vi "数据查询_数据查询.vi"() -> ()   [LabVIEW 2016]
uses:
  <vilib>/Utility/miscctls.llb/LVPointTypeDef.ctl
  <vilib>/addons/database/_DB Variant To Data/Database Variant To Data.xnode
panel:
  out "确定查询":bool
  out "显示项":string[](array[string])
  out "condition":string
  out "Line Chart":T1(xcontrol)
  in  "数据列表选择框":string(xcontrol)
  out "选中数据表":string
  in  "条件筛选":bool
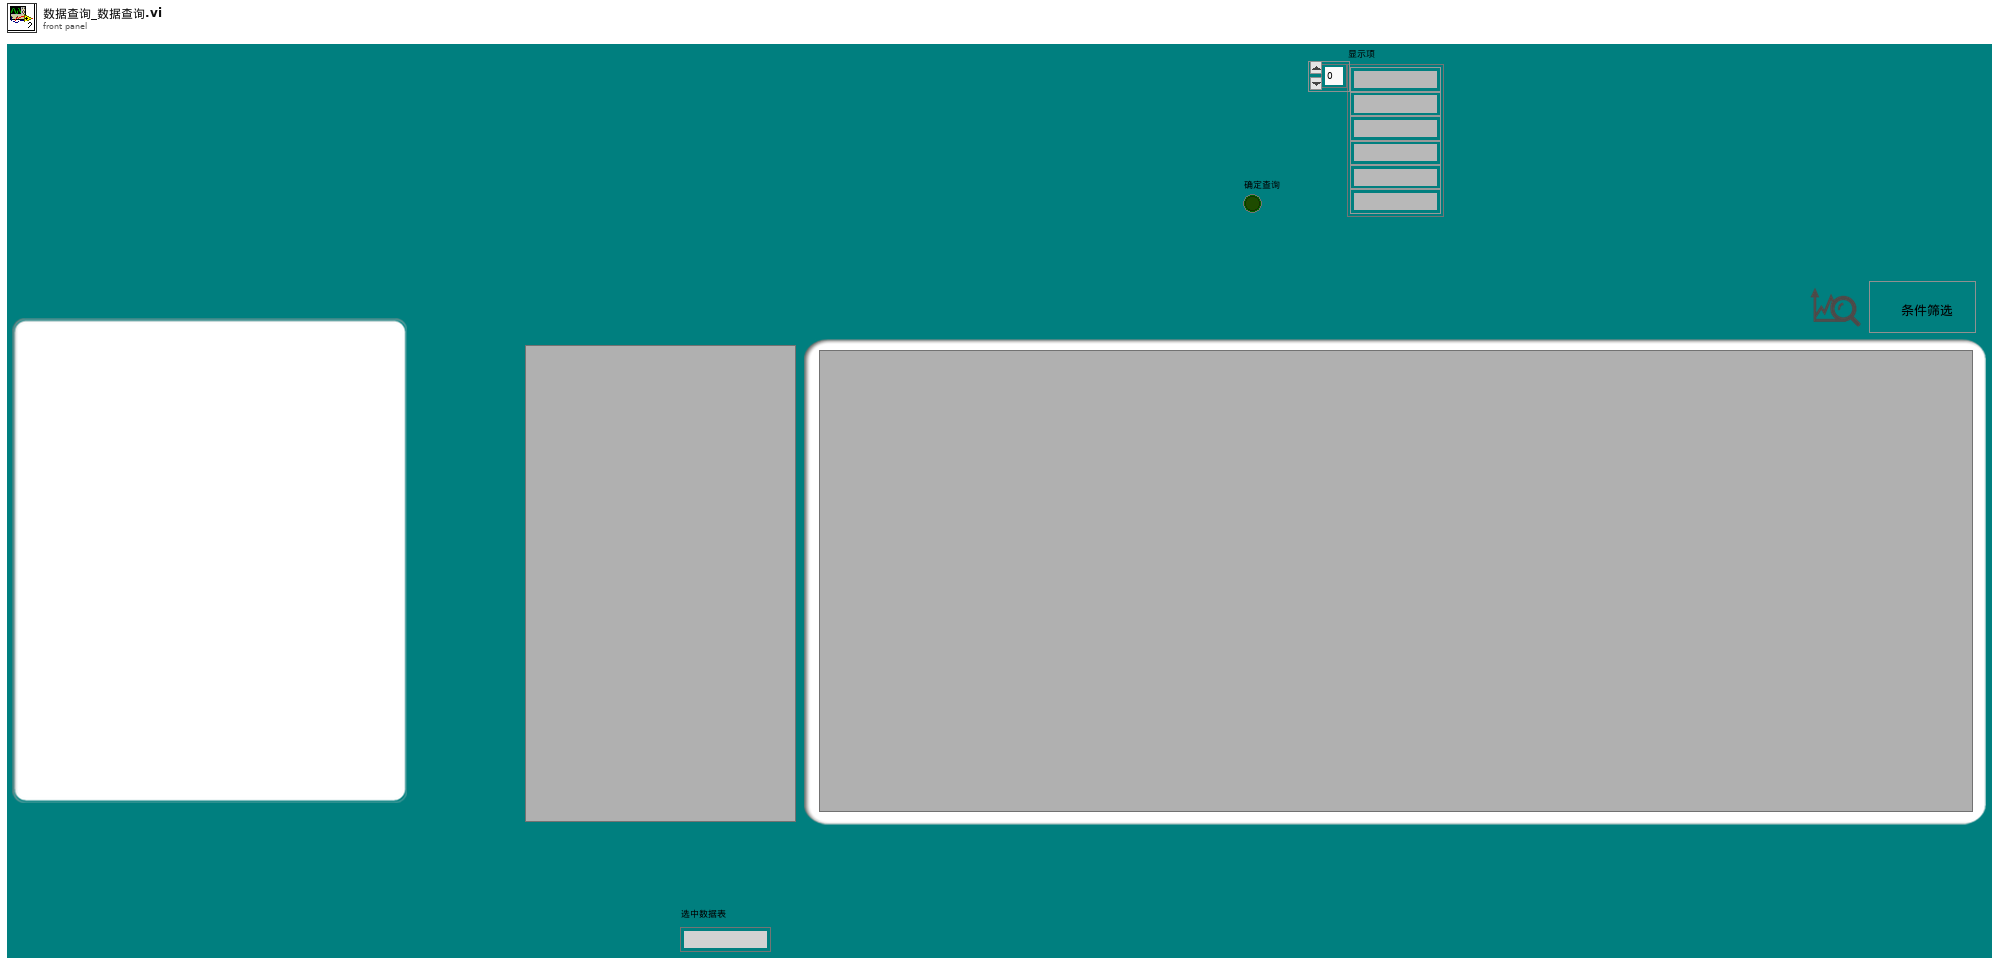
[diagram p1: front panel]
types:
  T1 = cluster{"X-Axis":string[], "Plots":cluster{"Data":dbl[], "Label":string, "Y-Axis":enum16{"Y-Axis 1", "Y-Axis 2", "Y-Axis 3", "Y-Axis 4", "Y-Axis 5", "Y-Axis 6", "Y-Axis 7", "Y-Axis 8", "Y-Axis 9", "Y-Axis 10"}, "Color":u32}[], "Plot Title":string}
  T2 = typedef "LVPointTypeDef.ctl" = cluster{"Horizontal":i16, "Vertical":i16}
  T3 = cluster{"Data":dbl[], "Label":string, "Y-Axis":enum16{"Y-Axis 1", "Y-Axis 2", "Y-Axis 3", "Y-Axis 4", "Y-Axis 5", "Y-Axis 6", "Y-Axis 7", "Y-Axis 8", "Y-Axis 9", "Y-Axis 10"}, "color":u32}
  T4 = cluster{"Data":dbl[], "Label":string, "Y-Axis":enum16{"Y-Axis 1", "Y-Axis 2", "Y-Axis 3", "Y-Axis 4", "Y-Axis 5", "Y-Axis 6", "Y-Axis 7", "Y-Axis 8", "Y-Axis 9", "Y-Axis 10"}, "Color":u32}
  T5 = cluster{"Data":dbl[], "Label":string, "Y-Axis":enum16{"Y-Axis 1", "Y-Axis 2", "Y-Axis 3", "Y-Axis 4", "Y-Axis 5", "Y-Axis 6", "Y-Axis 7", "Y-Axis 8", "Y-Axis 9", "Y-Axis 10"}, "color":u32}[]
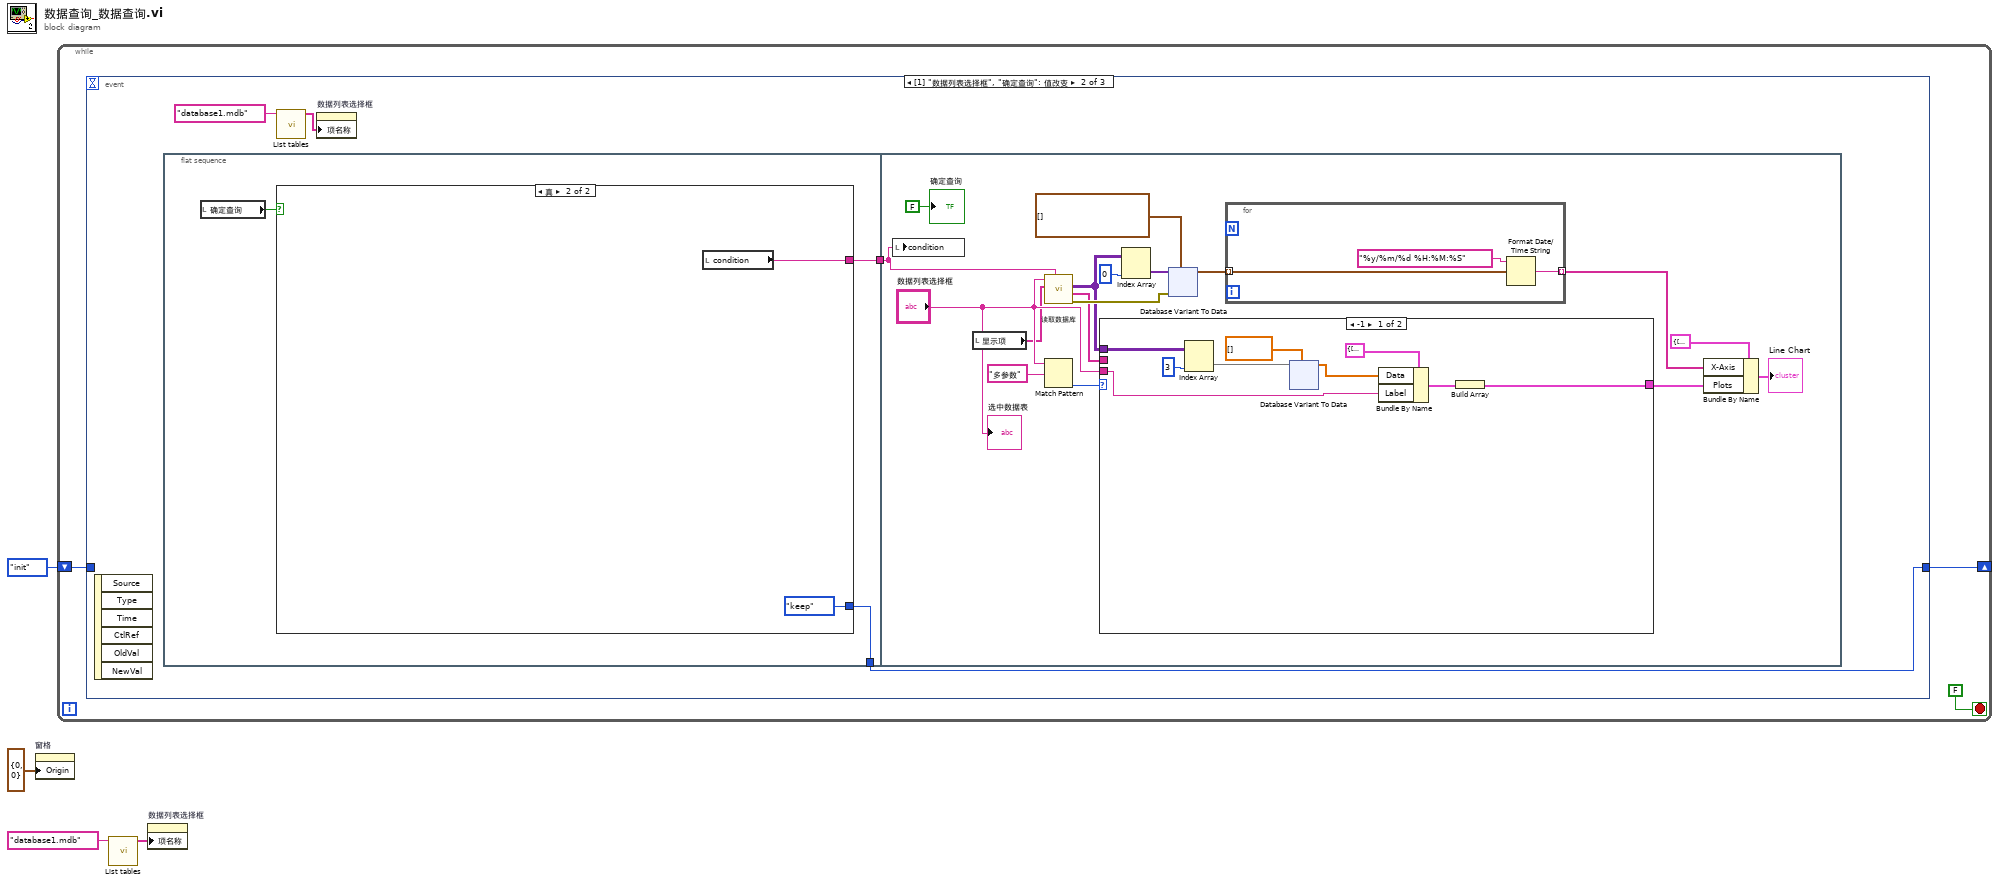
[diagram p0: block diagram]
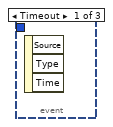
[diagram p2: hidden frame]
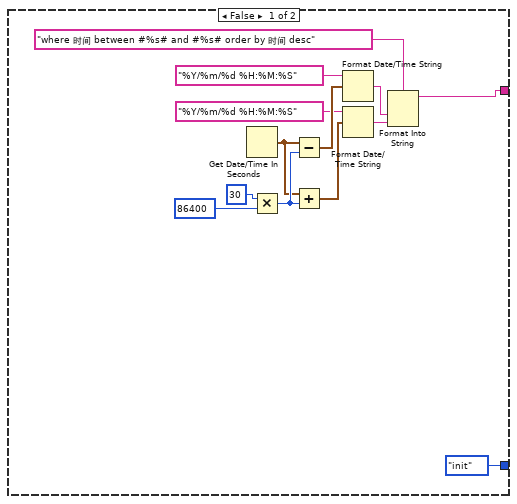
[diagram p3: hidden frame]
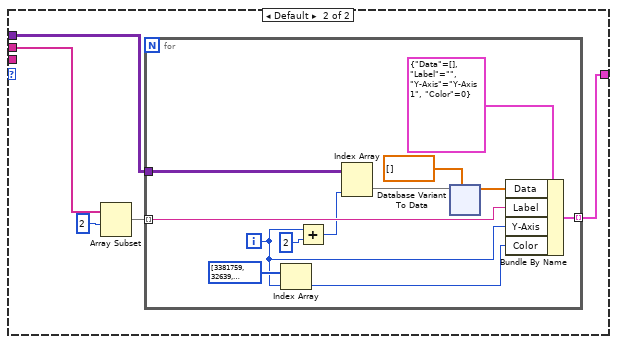
[diagram p4: hidden frame]
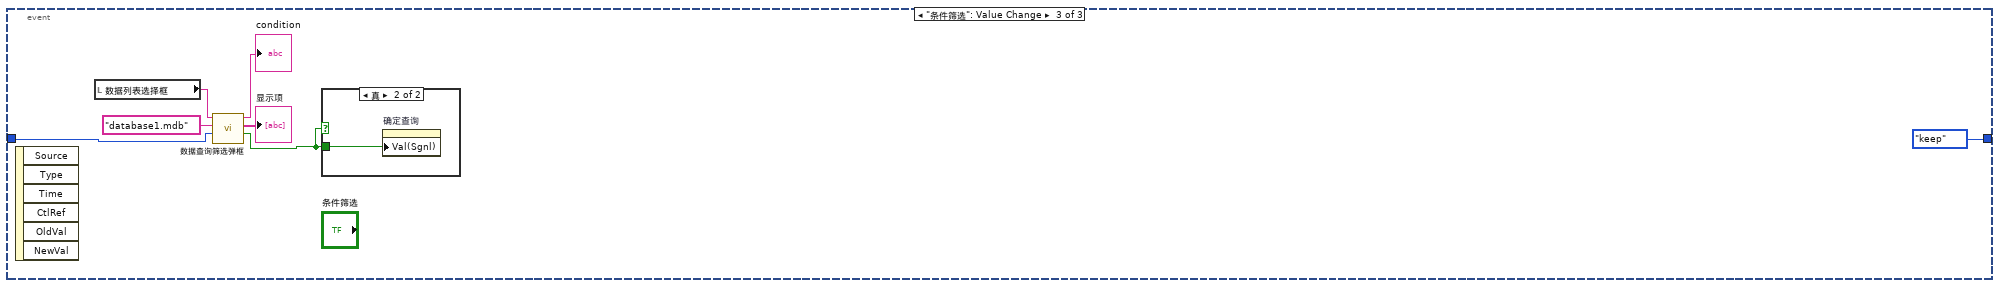
[diagram p5: hidden frame]
diagram:
  n1 = property on="窗格" class="Pane"("Origin"=T2 {"Horizontal"=0, "Vertical"=0} ("原点")) -> ()  [unwired: 2 in, 2 out]
  n2 = while {
    shift-right: [w5] -> _
    shift-left: enum16{"init", "keep"}."init" ("是否初始化") -> [w6]
    stop <- FALSE stop-if-true
    n3 = event shown="[1] \"数据列表选择框\", \"确定查询\": 值改变" {
      selector: _ -> [_ _ _]
      dyn-events: _ -> [_ _ _]
      timeout: _ -> [_ _ _]
      tunnel: w6 -> [_ _ w206]
      tunnel: [_ w8 enum16{"init", "keep"}."keep" ("是否初始化")] -> w5
      event Timeout {
        n4 = event-data() -> ()  [unwired: 1 in, 3 out]
      }
      event "数据列表选择框", "确定查询": Value Change {
        n5 = event-data() -> ()  [unwired: 1 in, 6 out]
        n6 = flat-sequence {
          tunnel: [w13] -> w9
          tunnel: [w12] -> w8
          tunnel: w9 -> [w30]
          frame #0 {
            n7 = local read "确定查询"() -> (w14:bool)
            n8 = case shown="真" w14 {
              tunnel: [w16 w28] -> w13
              tunnel: [enum16{"init", "keep"}."init" ("是否初始化") enum16{"init", "keep"}."keep" ("是否初始化")] -> w12
              frame False {
                n9 = Get Date/Time In Seconds() -> (seconds since 1Jan1904=w17:timestamp)
                n10 = Multiply(x=30, y=86400) -> (x*y=w18:i32)
                n11 = Subtract(x=w17, y=w18) -> (x-y=w24:timestamp)
                n12 = Add(x=w17, y=w18) -> (x+y=w23:timestamp)
                n13 = Format Date/Time String(time format string (%c)="%Y/%m/%d %H:%M:%S" ("时间格式字符串(%c)"), seconds (now)=w24) -> (date/time string=w26:string)  [unwired: 1 in]
                n14 = Format Date/Time String(time format string (%c)="%Y/%m/%d %H:%M:%S" ("时间格式字符串(%c)"), seconds (now)=w23) -> (date/time string=w27:string)  [unwired: 1 in]
                n15 = Format Into String(format string="where 时间 between #%s# and #%s# order by 时间 desc", w26, w27) -> (resulting string=w16:string)  [unwired: 2 in, 1 out]
              }
              frame True {
                n16 = local read "condition"() -> (w28:string)
              }
            }
          }
          frame #1 {
            n17 = local write "condition"(w30) -> ()
            n18 = local read "显示项"() -> (w32:string[])
            n19 = call "读取数据库.vi"("condition"=w30, "显示项"=w32, "组合框"="数据列表选择框") -> ("error out"=w43:errorcluster, "columns"=w35:string[], "data"=w42:variant[][])  [unwired: 5 in, 1 out]
            n20 = Match Pattern(string="数据列表选择框", regular expression="多参数" ("正则表达式")) -> (offset past match=w36:i32)  [unwired: 1 in, 3 out]
            n21 = case shown="-1" w36 {
              tunnel: w42 -> [w55 w98]
              tunnel: [w49 w94] -> w39
              tunnel: "数据列表选择框" -> [w48 _]
              tunnel: w35 -> [_ w97]
              frame -1 {
                n22 = Index Array(array=w55, index (col)=3 ("禁用的索引 (列)")) -> (element=w53:variant[])  [unwired: 1 in]
                n23 = xnode "Database Variant To Data"("database variant"=w53, "type"=sgl[] []) -> ("data"=w51:sgl[])  [unwired: 1 in, 1 out]
                n24 = Bundle By Name(cluster=T3 {"Data"=[], "Label"="", "Y-Axis"=enum."Y-Axis 1", "color"=3381759} ("Plot"), "Data"=w51, "Label"=w48) -> (w50:T3)
                n25 = Build Array(w50) -> (w49:T5)
              }
              frame Default {
                n26 = Array Subset(array=w97, index=2 ("索引")) -> (w95:string[])  [unwired: 1 in]
                n27 = for {
                  tunnel: w98 -> [w110]
                  tunnel: [w106] -> w94 mode=indexing
                  tunnel: w95 -> [w105] mode=indexing
                  i -> [w99]
                  n28 = Index Array(array=u32[] [3381759, 32639, 16744576, 16776960, 16711680, 16860, 8388863, 8404992, 10654332, 12819898], index=w99) -> (element=w101:u32)
                  n29 = Add(x=w99, y=2) -> (x+y=w103:i32)
                  n30 = Index Array(array=w110, index (col)=w103) -> (element=w109:variant[])  [unwired: 1 in]
                  n31 = xnode "Database Variant To Data"("database variant"=w109, "type"=sgl[] []) -> ("data"=w107:sgl[])  [unwired: 1 in, 1 out]
                  n32 = Bundle By Name(cluster=T4 {"Data"=[], "Label"="", "Y-Axis"=enum."Y-Axis 1", "Color"=0} ("Plot"), "Data"=w107, "Label"=w105, "Y-Axis"=w99, "Color"=w101) -> (w106:T4)
                }
              }
            }
            n33 = Index Array(array=w42, index (col)=0 ("禁用的索引 (列)")) -> (element=w45:variant[])  [unwired: 1 in]
            n34 = xnode "Database Variant To Data"("database variant"=w45, "error in (no error)"=w43, "type"=timestamp[] []) -> ("data"=w41:timestamp[])  [unwired: 1 out]
            n35 = for {
              tunnel: w41 -> [w151] mode=indexing
              tunnel: [w150] -> w40 mode=indexing
              n36 = Format Date/Time String(time format string (%c)="%y/%m/%d %H:%M:%S" ("时间格式字符串(%c)"), seconds (now)=w151) -> (date/time string=w150:string)  [unwired: 1 in]
            }
            n37 = Bundle By Name(cluster=T1 {"X-Axis"=[], "Plots"=[], "Plot Title"=""} ("Line Chart"), "X-Axis"=w40, "Plots"=w39) -> (→"Line Chart":T1)
            "选中数据表" <- "数据列表选择框"
            "确定查询" <- FALSE ("确定查询")
          }
        }
        n38 = call "List tables.vi"("database"="database1.mdb") -> ("tables"=w10:string[])  [unwired: 9 in, 1 out]
        n39 = property on="数据列表选择框" class="数据列表选择框 (严格)"("项名称"=w10) -> ()  [unwired: 2 in, 2 out]
      }
      event "条件筛选": Value Change {
        n40 = event-data() -> ()  [unwired: 1 in, 6 out]
        n41 = local read "数据列表选择框"() -> (w208:string)
        n42 = call "数据查询筛选弹框.vi"("是否初始化"=w206, "database"="database1.mdb", "table"=w208) -> ("确定输出"=w205:bool, "显示项"=→"显示项":string[], "condition"=→"condition":string)  [unwired: 5 in, 1 out]
        n43 = case shown="真" w205 {
          tunnel: w205 -> [_ w211]
          frame False {
          }
          frame True {
            n44 = property on="确定查询" class="Bool (严格)"("Val(Sgnl)"=w211) -> ()  [unwired: 2 in, 2 out]
          }
        }
      }
    }
  }
  n45 = call "List tables.vi"("database"="database1.mdb") -> ("tables"=w2:string[])  [unwired: 9 in, 1 out]
  n46 = property on="数据列表选择框" class="数据列表选择框 (严格)"("项名称"=w2) -> ()  [unwired: 2 in, 2 out]
